vi "Test Executive.vi"() -> ()   [LabVIEW 2020]
uses:
  Library - Test Executive.llb/Test Executive - Globals.vi
panel:
  in  "Help":bool
  in  "Calibration":bool
  in  "Manual Control":bool
  in  "Sequence Tab":bool
  out "Abort":bool
  out "Error":bool
  out "Running":bool
  in  "Tab Control":enum32{"TS", "M", "C", "H"}(tab)
  in  "Comment":string
  in  "Serial Number":string
  out "Sequence":string
  out "Report Text":string
  in  "Operator":string
  in  "Save Report":bool
  in  "Clear Report Text":bool
  out "Sequence Name":string="None"
  in  "Abort Button":bool
  in  "Sequence Run":bool
  in  "Sequence Load":bool
  out "Help Text":string="This is some help text\n"
  in  "Quit":bool
  # "Sequence"
  # "Progress"
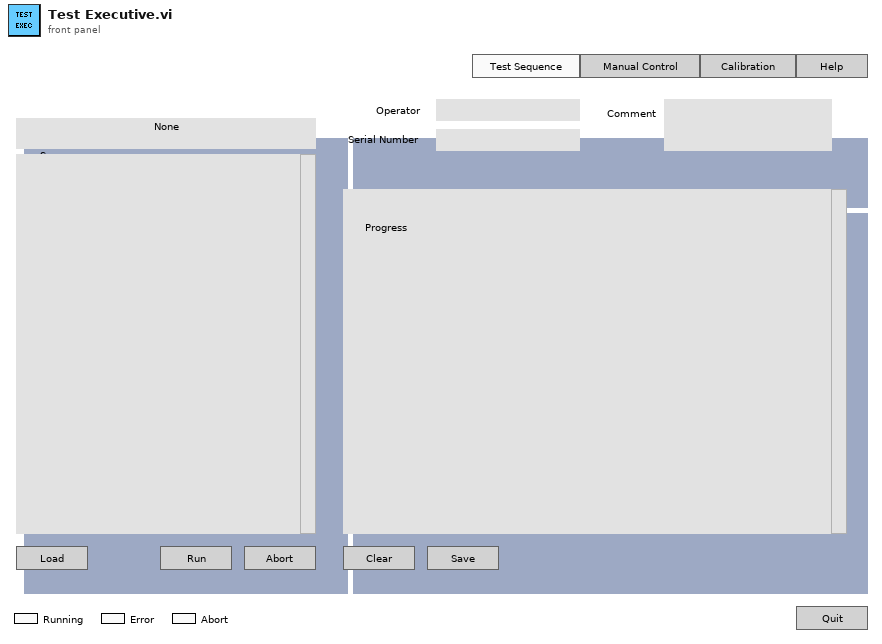
[diagram p1: front panel]
types:
  T1 = cluster{"Operator":string, "Serial Number":string, "Comment":string}
  T2 = cluster{"Operator Name":string, "UUT Serial Number":string, "Comment":string}
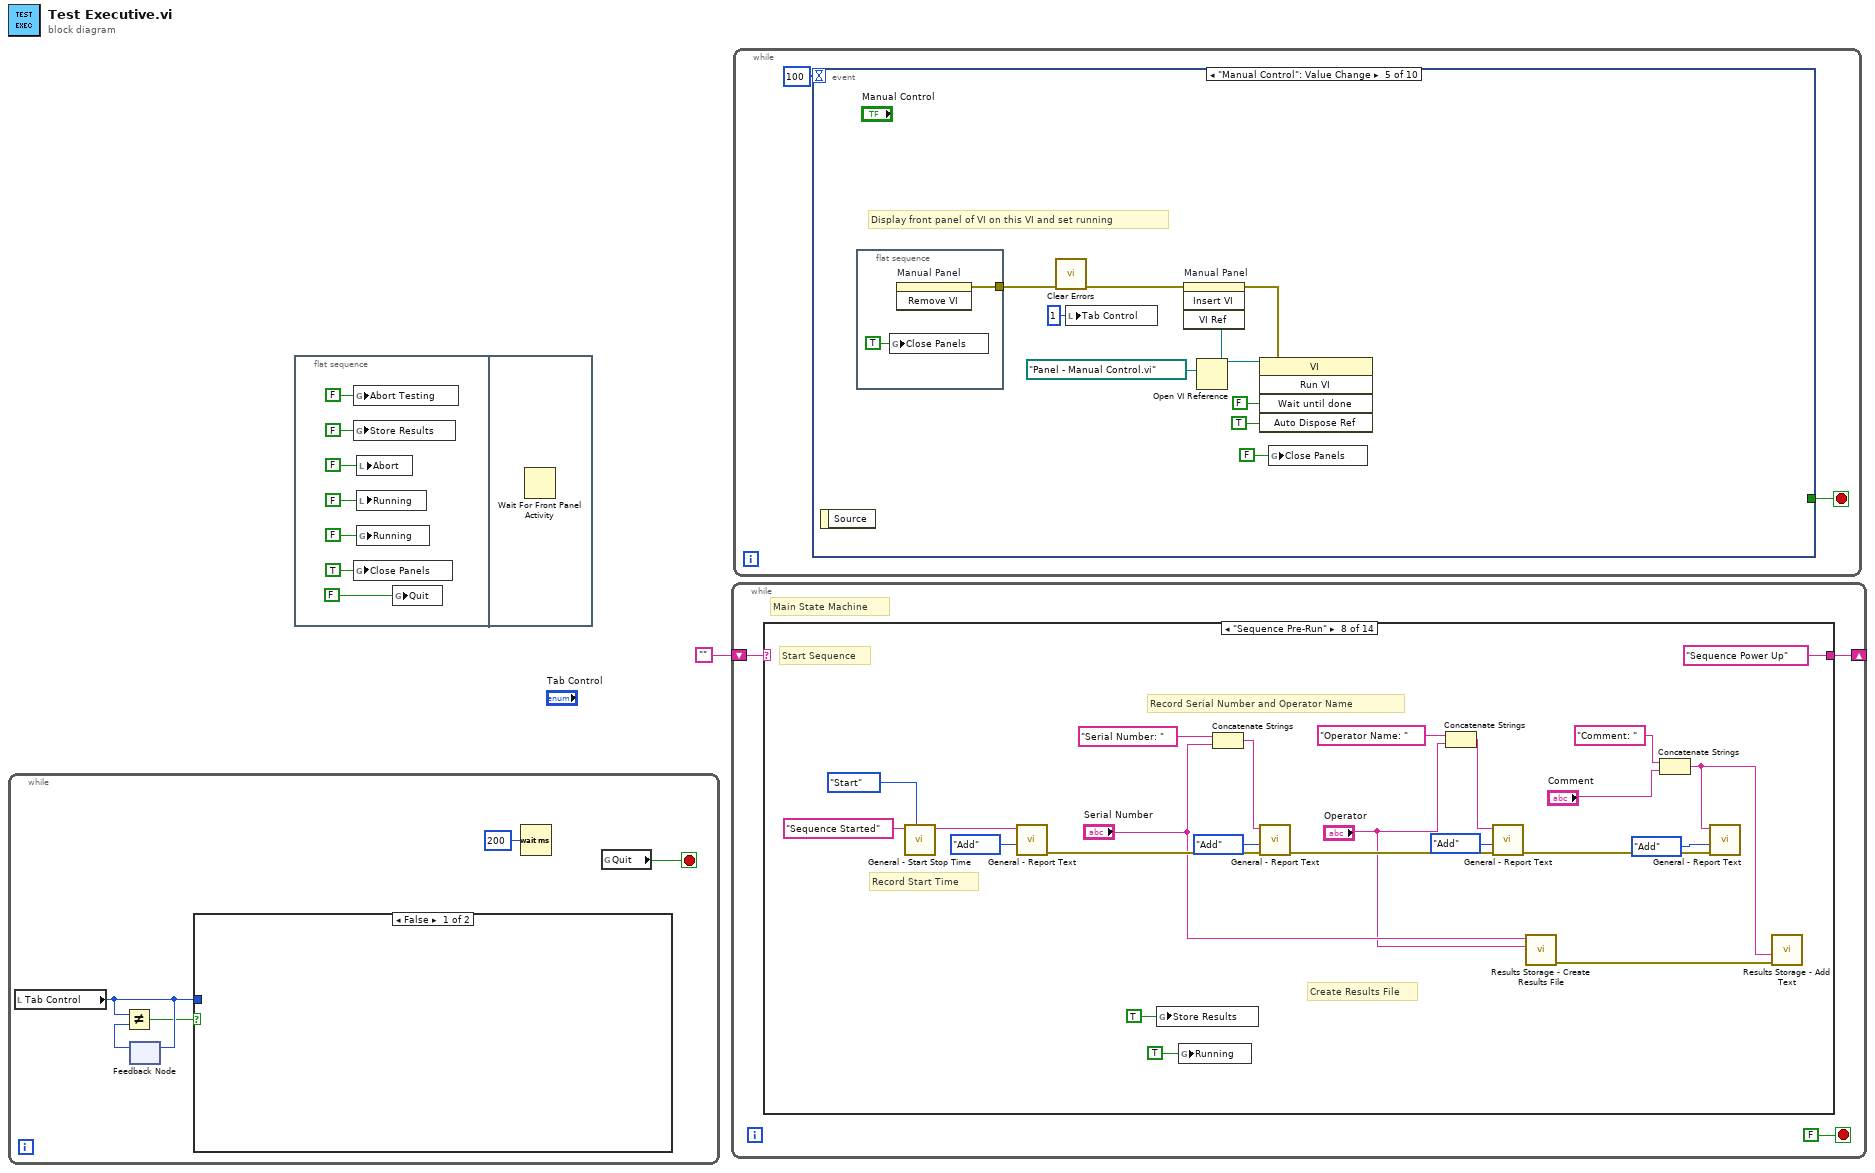
[diagram p0: block diagram]
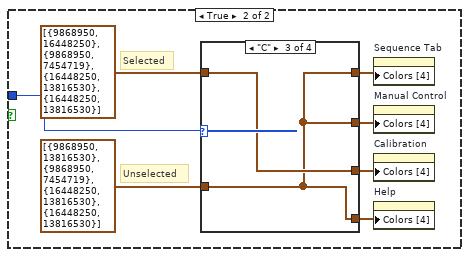
[diagram p2: hidden frame]
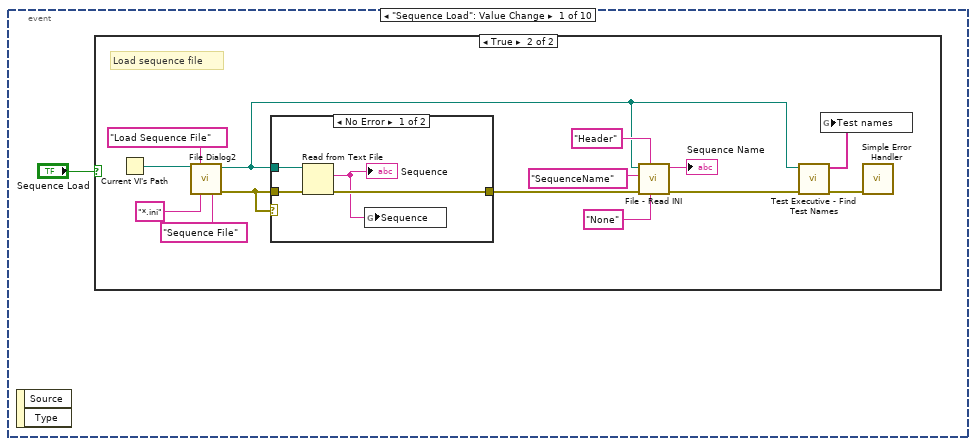
[diagram p6: hidden frame]
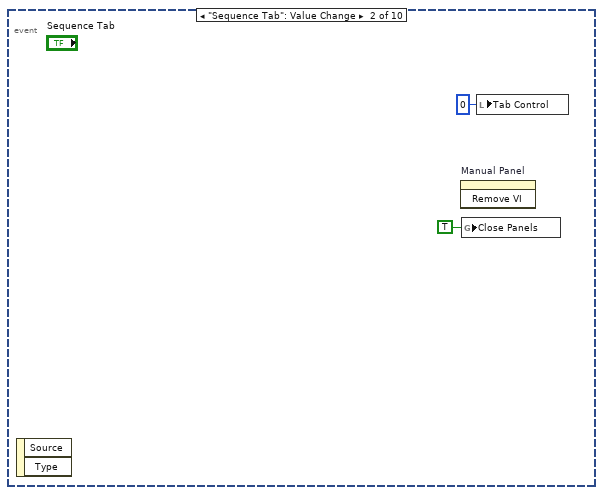
[diagram p9: hidden frame]
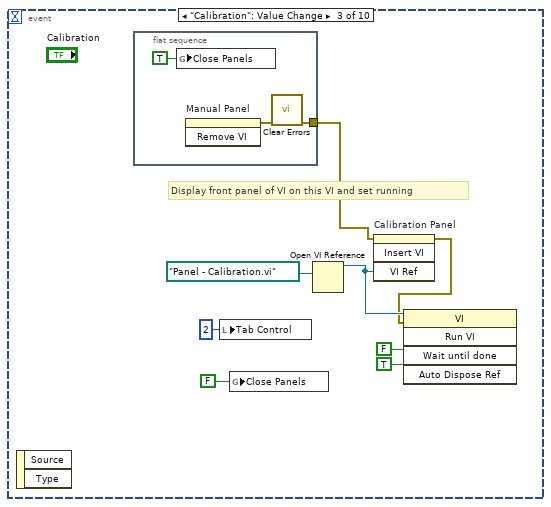
[diagram p10: hidden frame]
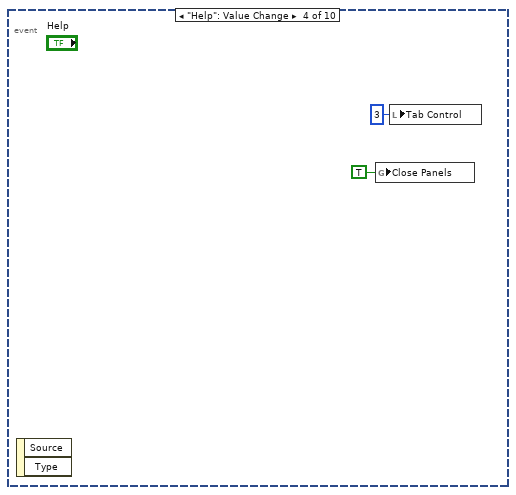
[diagram p11: hidden frame]
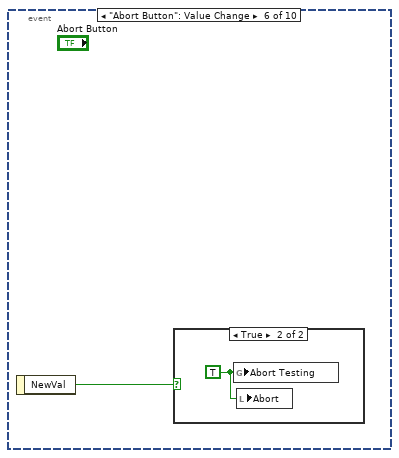
[diagram p12: hidden frame]
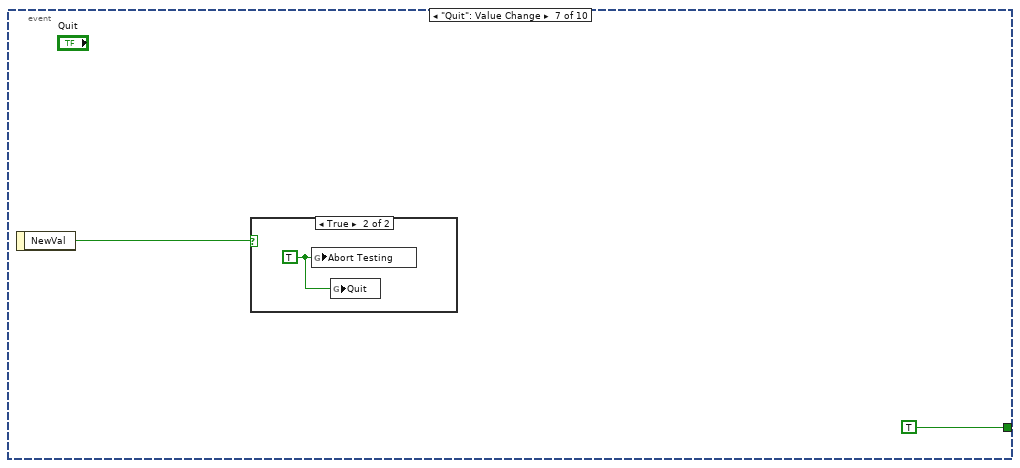
[diagram p14: hidden frame]
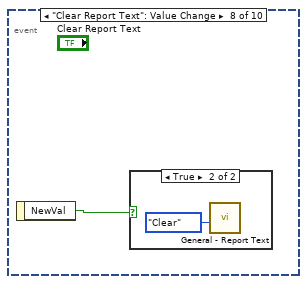
[diagram p16: hidden frame]
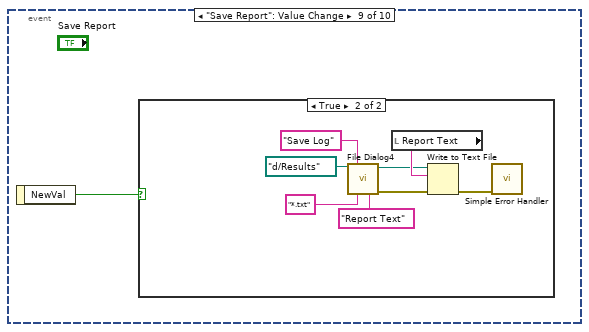
[diagram p18: hidden frame]
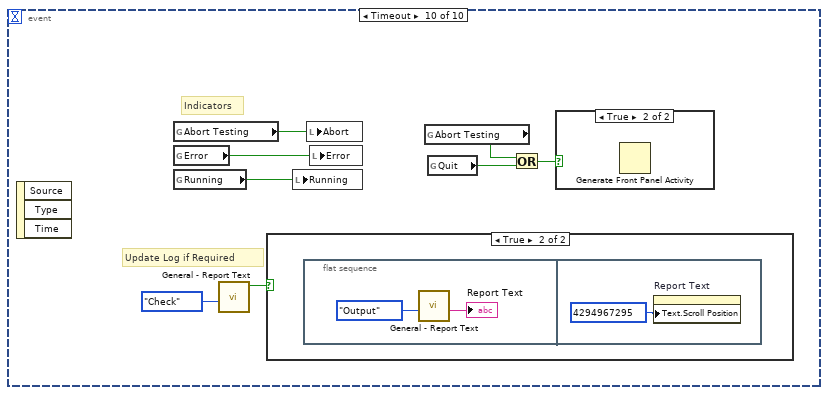
[diagram p20: hidden frame]
diagram:
  n1 = while {
    stop <- w3 stop-if-true
    n2 = local read "Tab Control"() -> (w6:enum32{"TS", "M", "C", "H"})
    n3 = feedback #1() -> (w4:enum32{"TS", "M", "C", "H"})  [unwired: 1 in]
    n4 = Not Equal?(x=w6, y=w4) -> (x != y?=w5:bool)
    n5 = feedback-in #1(w6) -> ()
    n6 = case shown="False" w5 {
      tunnel: w6 -> [_ w13]
      frame False {
      }
      frame True {
        # "Unselected"
        # "Selected"
        n7 = case shown="\"C\"" w13 {
          tunnel: cluster{u32, u32}[] [{9868950, 16448250}, {9868950, 7454719}, {16448250, 13816530}, {16448250, 13816530}] ("Colors [4]") -> [w15 w17 w19 w21]
          tunnel: cluster{u32, u32}[] [{9868950, 13816530}, {9868950, 7454719}, {16448250, 13816530}, {16448250, 13816530}] ("Colors [4]") -> [w14 w16 w18 w20]
          tunnel: [w15 w16 w18 w20] -> w10
          tunnel: [w14 w17 w18 w20] -> w9
          tunnel: [w14 w16 w19 w20] -> w8
          tunnel: [w14 w16 w18 w21] -> w7
          frame "TS", Default {
          }
          frame "M" {
          }
          frame "C" {
          }
          frame "H" {
          }
        }
        n8 = property on="Sequence Tab" class="Bool"("Colors [4]"=w10) -> ()  [unwired: 2 in, 2 out]
        n9 = property on="Manual Control" class="Bool"("Colors [4]"=w9) -> ()  [unwired: 2 in, 2 out]
        n10 = property on="Calibration" class="Bool"("Colors [4]"=w8) -> ()  [unwired: 2 in, 2 out]
        n11 = property on="Help" class="Bool"("Colors [4]"=w7) -> ()  [unwired: 2 in, 2 out]
      }
    }
    n12 = Wait (ms)(milliseconds to wait=u32 200) -> ()  [unwired: 1 out]
    n13 = global read "Test Executive - Globals.vi" "Quit"() -> (w3:bool)
  }
  n14 = flat-sequence {
    frame #0 {
      n15 = global write "Test Executive - Globals.vi" "Abort Testing"(FALSE ("Abort Testing")) -> ()
      n16 = global write "Test Executive - Globals.vi" "Store Results"(FALSE ("Abort Testing")) -> ()
      n17 = global write "Test Executive - Globals.vi" "Close Panels"(TRUE ("Close Panels")) -> ()
      n18 = local write "Abort"(FALSE ("Abort")) -> ()
      n19 = local write "Running"(FALSE ("Abort")) -> ()
      n20 = global write "Test Executive - Globals.vi" "Running"(FALSE ("Test Running")) -> ()
      n21 = global write "Test Executive - Globals.vi" "Quit"(FALSE ("Quit")) -> ()
    }
    frame #1 {
      n22 = Wait For Front Panel Activity() -> ()  [unwired: 3 in, 1 out]
    }
  }
  n23 = while {
    shift-right: [w30] -> _
    shift-left: "" -> [w31]
    stop <- FALSE stop-if-true
    # "Main State Machine"
    n24 = case shown="\"Sequence Pre-Run\"" w31 {
      tunnel: ["Idle" w58 w64 w65 w77 w115 "Sequence Pre-Run" ("f") "Sequence Power Up" ("f") "Sequence Running" ("f") "Sequence Power Down" ("f") "Sequence Pass Fail" ("f") "Sequence Store Results" ("f") "Idle" ("f") ""] -> w30
      frame "Start", Default {
        w34 = FALSE
        w35 = FALSE ("Running")
        # "Hide tab control (make transparent)"
        # "Auto Load Main Sequence"
        # "Load Help Text"
        # "Clear Indicators"
        # "Define File Paths"
        # "Define Test Equipment"
        n25 = disable-structure shown="Disabled" {
          frame Disabled {
            n26 = property class="VI" props=["Panel"]() -> (reference out=w46:refnum<vi>)  [unwired: 2 in, 2 out]
            n27 = call "Dialog Box - Resize Window.vi"("Height"=i16 493, "Width"=i16 900, "reference"=w46) -> ()  [unwired: 8 in, 1 out]
          }
          frame Enabled {
          }
        }
        n28 = call "Sequence - Define Test Equipment.vi"() -> ()  [unwired: 11 in, 1 out]
        n29 = global write "Test Executive - Globals.vi" "Abort Testing"(w34) -> ()
        n30 = global write "Test Executive - Globals.vi" "Error"(w34) -> ()
        n31 = global write "Test Executive - Globals.vi" "Running"(w34) -> ()
        n32 = global write "Test Executive - Globals.vi" "Quit"(w34) -> ()
        n33 = call "Test Executive - Define Paths.vi"() -> ()  [unwired: 12 in]
        n34 = call <vilib>:"Application Directory.vi"() -> ("Application Directory"=w36:path)
        n35 = property on="Tab Control" class="TabCtl (strict)"("Colors"=cluster{u32, u32} {16777216, 16777216}, "Tabs Visible?"=FALSE) -> ()  [unwired: 2 in, 2 out]
        n36 = Build Path(base path=w36, name or relative path="Help.txt") -> (appended path=w43:path)
        n37 = Build Path(base path=w36, name or relative path="Sequence - Main.ini") -> (appended path=w37:path)
        n38 = Read from Text File(file (use dialog)=w43) -> (text=w42:string, error out=w41:errorcluster)  [unwired: 3 in, 2 out]
        n39 = Read from Text File(file (use dialog)=w37) -> (text=w39:string, error out=w40:errorcluster)  [unwired: 3 in, 2 out]
        n40 = case shown="No Error" w41 {
          tunnel: w42 -> [w56 _]
          frame No Error {
            "Help Text" <- w56
          }
          frame Error {
          }
        }
        n41 = case shown="No Error" w40 {
          tunnel: w39 -> [w50 _]
          tunnel: w37 -> [w51 _]
          frame No Error {
            n42 = local write "Sequence"(w50) -> ()
            n43 = call "Test Executive - Find Test Names.vi"("Configuration File Path"=w51) -> ("Test Names"=w49:string[])  [unwired: 9 in, 1 out]
            n44 = global write "Test Executive - Globals.vi" "Test names"(w49) -> ()
            n45 = call "File - Read INI.vi"("Default String"="None", "Section"="Header", "Key"="SequenceName", "configuration file path"=w51) -> ("String"=w52:string)  [unwired: 6 in, 1 out]
            n46 = local write "Sequence Name"(w52) -> ()
            n47 = global write "Test Executive - Globals.vi" "Sequence"(w50) -> ()
          }
          frame Error {
          }
        }
        "Running" <- w35
        "Error" <- w35
        "Abort" <- w35
      }
      frame "Idle" {
        # "Wait For Front Panel Activity"
        n48 = global read "Test Executive - Globals.vi" "Quit"() -> (w60:bool)
        n49 = Select(t="Quit", s=w60, f="Sequence Controls") -> (s? t:f=w58:string)
      }
      frame "Sequence Controls" {
        # "Sequence Controls"
        n50 = Select(t="Sequence Check", s="Sequence Run", f="Idle") -> (s? t:f=w64:string)
      }
      frame "Sequence Check" {
        # "Check Sequence Name"
        # "Sequence Check"
        n51 = local read "Sequence Name"() -> (w67:string)
        n52 = Equal?(x=w67, y="None") -> (x = y?=w69:bool)
        n53 = case shown="True" w69 {
          tunnel: "Sequence Start" -> [w70 _]
          tunnel: [w70 "Idle"] -> w65
          frame False {
          }
          frame True {
            n54 = call "Dialog Box - One Button.vi"("Text"="ERROR: Sequence name is set to \"None\".") -> ()  [unwired: 10 in, 1 out]
          }
        }
      }
      frame "Sequence Start" {
        # "Start of Sequence"
        # "Configure Results Storage"
        n55 = local read "Serial Number"() -> (w87:string)
        n56 = call <vilib>:"Dflt Data Dir.vi"() -> ("App:Default Data Directory"=w90:path)
        n57 = local read "Comment"() -> (w85:string)
        n58 = local read "Operator"() -> (w88:string)
        n59 = Build Path(base path=w90, name or relative path="Results") -> (appended path=w91:path)
        n60 = call "General - Check if Mac.vi"() -> ("Mac"=w92:bool)  [unwired: 2 in]
        n61 = Path To String(path=w91) -> (string=w75:string)
        n62 = Bundle("Operator"=w88, "Serial Number"=w87, "Comment"=w85) -> (w86:T1)  [unwired: 1 in]
        n63 = case shown="False" w92 {
          tunnel: [w109 w113] -> w73
          tunnel: w75 -> [w107 w111]
          frame True {
            n64 = call "Test Executive - Sequence File Value.vi"("Default String"=w107, "Section (Current Test)"="results" ("Section"), "Key"="directorymac") -> ("String"=w109:string)  [unwired: 5 in, 3 out]
          }
          frame False {
            n65 = call "Test Executive - Sequence File Value.vi"("Default String"=w111, "Section (Current Test)"="results" ("Section"), "Key"="directorywin") -> ("String"=w113:string)  [unwired: 5 in, 3 out]
          }
        }
        n66 = disable-structure shown="Enabled" {
          disable-tunnel: w86 -> [w100 _]
          disable-tunnel: [w99 _] -> w84
          disable-tunnel: [w98 FALSE ("Cancel")] -> w78
          frame Disabled {
            n67 = call "Dialog Box - Test Details.vi"("Values In"=w100) -> ("Values Out"=w99:T2, "Cancel"=w98:bool)  [unwired: 7 in, 1 out]
          }
          frame Enabled {
          }
        }
        n68 = Unbundle By Name(w84) -> ("Operator Name"=w83:string, "UUT Serial Number"=w82:string, "Comment"=w81:string)
        n69 = call "General - Check if Linux.vi"() -> ("Linux"=w76:bool)  [unwired: 2 in]
        n70 = case shown="False" w76 {
          tunnel: [w104 w106] -> w74
          tunnel: w75 -> [w102 _]
          tunnel: w73 -> [_ w106]
          frame True {
            n71 = call "Test Executive - Sequence File Value.vi"("Default String"=w102, "Section (Current Test)"="results" ("Section"), "Key"="directorylinux") -> ("String"=w104:string)  [unwired: 5 in, 3 out]
          }
          frame False {
          }
        }
        n72 = local write "Serial Number"(w82) -> ()
        n73 = local write "Operator"(w83) -> ()
        n74 = local write "Comment"(w81) -> ()
        n75 = String To Path(string=w74) -> (path=w94:path)
        n76 = global write "Test Executive - Globals.vi" "Operator Name"(w83) -> ()
        n77 = global write "Test Executive - Globals.vi" "Serial Number"(w82) -> ()
        n78 = global write "Test Executive - Globals.vi" "Comment"(w81) -> ()
        n79 = global write "Test Executive - Globals.vi" "Results Directory"(w94) -> ()
        n80 = call "Results Storage - Setup.vi"("Rename Files on Close"=TRUE, "Results Directory"=w94) -> ()  [unwired: 9 in, 1 out]
        n81 = call "General - Report Text.vi"("Mode (Add)"=enum16{"Add", "Output", "Clear", "Check"}."Clear") -> ()  [unwired: 8 in, 3 out]
        n82 = global write "Test Executive - Globals.vi" "Abort Testing"(FALSE ("Abort Testing")) -> ()
        n83 = global write "Test Executive - Globals.vi" "Unit Passed"(FALSE ("Pass")) -> ()
        n84 = Select(t="Idle" ("f"), s=w78, f="Sequence Check Equipment") -> (s? t:f=w77:string)
      }
      frame "Sequence Check Equipment" {
        # "Check Test Equipment"
        # "Check Test Equipment"
        n85 = call "Sequence - Check Test Equipment.vi"() -> ("error out"=w118:errorcluster, "PASS"=w119:bool)  [unwired: 10 in]
        n86 = Not(x=w119) -> (.not. x?=w117:bool)
        n87 = case shown="False" w117 {
          tunnel: "Sequence Asset" -> [w120 _]
          tunnel: [w120 "Idle"] -> w115
          tunnel: w118 -> [_ _]
          frame False {
          }
          frame True {
            n88 = call "Dialog Box - One Button.vi"("Text"="ERROR: Test equipment check failed.") -> ()  [unwired: 10 in, 1 out]
          }
        }
      }
      frame "Sequence Asset" {
        # "Test Equipment is Defined is \"Sequence - Define Test Equipment.vi\""
        # "Enter Equipment Asset Numbers"
        n89 = global read "Test Executive - Globals.vi" "Asset Number Recording"() -> (w123:bool)
        n90 = case shown="True" w123 {
          frame False {
          }
          frame True {
            n91 = call "Test Equipment - Asset Numbers.vi"("Mode"=enum16{"Edit", "Define", "Load", "Save", "CSV"}."Load") -> ("error out"=w125:errorcluster)  [unwired: 9 in, 1 out]
            n92 = call "Test Equipment - Asset Numbers.vi"("error in (no error)"=w125, "Mode"=enum16{"Edit", "Define", "Load", "Save", "CSV"}."Edit") -> ("error out"=w126:errorcluster)  [unwired: 8 in, 1 out]
            n93 = call "Test Equipment - Asset Numbers.vi"("error in (no error)"=w126, "Mode"=enum16{"Edit", "Define", "Load", "Save", "CSV"}."Save") -> ()  [unwired: 8 in, 2 out]
          }
        }
      }
      frame "Sequence Pre-Run" {
        # "Create Results File"
        # "Record Serial Number and Operator Name"
        # "Record Start Time"
        # "Start Sequence"
        n94 = call "General - Start Stop Time.vi"("Start / Stop (Start)"=enum16{"Start", "Stop"}."Start", "Initial String"="Sequence Started") -> ("String with Time / Date"=w150:string)  [unwired: 8 in, 1 out]
        n95 = call "General - Report Text.vi"("Mode (Add)"=enum16{"Add", "Output", "Clear", "Check"}."Add", "Text In"=w150) -> ("error out"=w141:errorcluster)  [unwired: 7 in, 2 out]
        n96 = global write "Test Executive - Globals.vi" "Store Results"(TRUE ("Store Results")) -> ()
        n97 = global write "Test Executive - Globals.vi" "Running"(TRUE ("Test Running")) -> ()
        n98 = Concatenate Strings("Serial Number: " ("string"), "Serial Number") -> (w146:string)
        n99 = call "General - Report Text.vi"("error in (no error)"=w141, "Mode (Add)"=enum16{"Add", "Output", "Clear", "Check"}."Add", "Text In"=w146) -> ("error out"=w140:errorcluster)  [unwired: 6 in, 2 out]
        n100 = Concatenate Strings("Operator Name: " ("string"), "Operator") -> (w143:string)
        n101 = call "General - Report Text.vi"("error in (no error)"=w140, "Mode (Add)"=enum16{"Add", "Output", "Clear", "Check"}."Add", "Text In"=w143) -> ("error out"=w132:errorcluster)  [unwired: 6 in, 2 out]
        n102 = call "Results Storage - Create Results File.vi"("Operator Name"="Operator", "Serial Number"="Serial Number") -> ("error out"=w131:errorcluster)  [unwired: 9 in]
        n103 = Concatenate Strings("Comment: " ("string"), "Comment") -> (w130:string)
        n104 = call "General - Report Text.vi"("error in (no error)"=w132, "Mode (Add)"=enum16{"Add", "Output", "Clear", "Check"}."Add", "Text In"=w130) -> ()  [unwired: 6 in, 3 out]
        n105 = call "Results Storage - Add Text.vi"("error in (no error)"=w131, "Text"=w130) -> ()  [unwired: 9 in, 1 out]
      }
      frame "Sequence Power Up" {
        # "Reset all Test Equipment then Power Up Unit Under Test"
        # "Sequence Power Up"
        n106 = call "Sequence - Reset All.vi"() -> ("error out"=w157:errorcluster)  [unwired: 11 in]
        n107 = call "Test Executive - Display Error.vi"("Clear Error"=TRUE, "error in (no error)"=w157) -> ("error out"=w156:errorcluster)  [unwired: 9 in]
        n108 = call "Sequence - Power Up.vi"("error in (no error)"=w156) -> ("error out"=w155:errorcluster)  [unwired: 10 in]
        n109 = call "Test Executive - Display Error.vi"("Clear Error"=TRUE, "error in (no error)"=w155) -> ()  [unwired: 9 in, 1 out]
      }
      frame "Sequence Running" {
        # "Run Sequence"
        n110 = global read "Test Executive - Globals.vi" "Test names"() -> (w159:string[])
        n111 = for {
          tunnel: w159 -> [w162] mode=indexing
          stop <- w163 stop-if-true
          # "Step Through Each Test"
          n112 = call "Sequence - Action Test.vi"("Test"=w162) -> ("error out"=w161:errorcluster)  [unwired: 10 in]
          n113 = stacked-sequence {
            tunnel: [w166] -> w163
            tunnel: w161 -> [w165]
            frame #0 {
              n114 = call "Test Executive - Display Error.vi"("error in (no error)"=w165) -> ("error out"=w164:errorcluster)  [unwired: 10 in]
              n115 = Unbundle By Name(w164) -> ("status"=w167:bool)
              n116 = global read "Test Executive - Globals.vi" "Abort Testing"() -> (w166:bool)
              n117 = local write "Error"(w167) -> ()
            }
          }
        }
      }
      frame "Sequence Power Down" {
        # "Power Down Unit Under Test then Reset all Test Equipment"
        # "Sequence Power Down"
        n118 = call "Sequence - Power Down.vi"() -> ("error out"=w168:errorcluster)  [unwired: 11 in]
        n119 = call "Test Executive - Display Error.vi"("Clear Error"=TRUE, "error in (no error)"=w168) -> ("error out"=w169:errorcluster)  [unwired: 9 in]
        n120 = call "Sequence - Reset All.vi"("error in (no error)"=w169) -> ("error out"=w170:errorcluster)  [unwired: 10 in]
        n121 = call "Test Executive - Display Error.vi"("Clear Error"=TRUE, "error in (no error)"=w170) -> ()  [unwired: 9 in, 1 out]
      }
      frame "Sequence Pass Fail" {
        # "Add Stop Time"
        # "Sequence Pass / Fail"
        # "Display Banner"
        # "Pass / Fail ??"
        n122 = call "General - Report Text.vi"("Mode (Add)"=enum16{"Add", "Output", "Clear", "Check"}."Output") -> ("Report Text Out"=w183:string)  [unwired: 8 in, 2 out]
        n123 = Search/Split String(string=w183, search string/char (-)="ERROR") -> (offset of match=w203:i32)  [unwired: 1 in, 2 out]
        n124 = Search/Split String(string=w183, search string/char (-)="FAIL") -> (offset of match=w197:i32)  [unwired: 1 in, 2 out]
        n125 = Search/Split String(string=w183, search string/char (-)="PASS") -> (offset of match=w184:i32)  [unwired: 1 in, 2 out]
        n126 = Greater Than 0?(x=w203) -> (x > 0?=w204:bool)
        n127 = Greater Than 0?(x=w197) -> (x > 0?=w198:bool)
        n128 = Greater Than 0?(x=w184) -> (x > 0?=w181:bool)
        n129 = Select(t="UNIT PASSED", s=w181, f="UNIT FAILED") -> (s? t:f=w180:string)
        n130 = Select(t="UNIT FAILED", s=w198, f=w180) -> (s? t:f=w205:string)
        n131 = global read "Test Executive - Globals.vi" "Abort Testing"() -> (w175:bool)
        n132 = Select(t="UNIT FAILED (ERRORS)", s=w204, f=w205) -> (s? t:f=w178:string)
        n133 = Select(t="TESTING ABORTED", s=w175, f=w178) -> (s? t:f=w176:string)
        n134 = Select(t="Sequence Aborted", s=w175, f="Sequence Completed" ("Initial String")) -> (s? t:f=w192:string)
        n135 = call "General - Report Text.vi"("Mode (Add)"=enum16{"Add", "Output", "Clear", "Check"}."Add", "Text In"=w176) -> ("error out"=w188:errorcluster)  [unwired: 7 in, 2 out]
        n136 = call "General - Start Stop Time.vi"("Start / Stop (Start)"=enum16{"Start", "Stop"}."Stop", "Initial String"=w192) -> ("String with Time / Date"=w190:string)  [unwired: 8 in, 1 out]
        n137 = Equal?(x="UNIT PASSED", y=w176) -> (x = y?=w174:bool)
        n138 = global write "Test Executive - Globals.vi" "Unit Passed"(w174) -> ()
        n139 = call "Dialog Box - Pass Fail Banner.vi"("Pass"=w174, "Text"=w176) -> ()  [unwired: 9 in, 1 out]
        n140 = call "General - Report Text.vi"("error in (no error)"=w188, "Mode (Add)"=enum16{"Add", "Output", "Clear", "Check"}."Add", "Text In"=w190) -> ()  [unwired: 6 in, 3 out]
      }
      frame "Sequence Store Results" {
        # "Record Asset Numbers"
        # "Sequence Store Results"
        # "Close Results File"
        n141 = global read "Test Executive - Globals.vi" "Asset Number Recording"() -> (w209:bool)
        n142 = global read "Test Executive - Globals.vi" "Unit Passed"() -> (w206:bool)
        n143 = case shown="True" w209 {
          tunnel: [_ w217] -> w208
          frame False {
          }
          frame True {
            n144 = call "Test Equipment - Asset Numbers.vi"("Mode"=enum16{"Edit", "Define", "Load", "Save", "CSV"}."CSV") -> ("Output"=w218:string)  [unwired: 9 in, 1 out]
            n145 = call "Results Storage - Add Text.vi"("Add New Line (True)"=FALSE, "Text"=w218) -> ("error out"=w217:errorcluster)  [unwired: 9 in]
          }
        }
        n146 = global read "Test Executive - Globals.vi" "Abort Testing"() -> (w207:bool)
        n147 = Select(t=enum16{"auto", "passed", "failed", "aborted"}."passed" ("Result (auto)"), s=w206, f=enum16{"auto", "passed", "failed", "aborted"}."failed" ("Result (auto)")) -> (s? t:f=w211:enum16{"auto", "passed", "failed", "aborted"})
        n148 = Select(t=enum16{"auto", "passed", "failed", "aborted"}."aborted" ("Result (auto)"), s=w207, f=w211) -> (s? t:f=w210:enum16{"auto", "passed", "failed", "aborted"})
        n149 = call "Results Storage - Close Results File.vi"("error in (no error)"=w208, "Result (auto)"=w210) -> ()  [unwired: 9 in, 1 out]
      }
      frame "Quit" {
        # "Exit Program"
        n150 = flat-sequence {
          frame #0 {
            # "Exit completely if\ncompiled"
            n151 = call "General - Check if EXE.vi"() -> ("EXE"=w221:bool)  [unwired: 2 in]
            n152 = global write "Test Executive - Globals.vi" "Close Panels"(TRUE ("Close Panels")) -> ()
            n153 = Quit LabVIEW(quit? (T)=w221) -> ()
          }
          frame #1 {
            # "Make tab control visible"
            n154 = property on="Tab Control" class="TabCtl (strict)"("Colors"=cluster{u32, u32} {7171459, 7171459}, "Tabs Visible?"=TRUE) -> ()  [unwired: 2 in, 2 out]
          }
          frame #2 {
            n155 = Stop() -> ()  [unwired: 1 in]
          }
        }
      }
    }
  }
  n156 = while {
    stop <- w225 stop-if-true
    n157 = event shown="[4] \"Manual Control\": Value Change" {
      selector: _ -> [_ _ _ _ _ _ _ _ _ _]
      dyn-events: _ -> [_ _ _ _ _ _ _ _ _ _]
      timeout: 100 -> [_ _ _ _ _ _ _ _ _ _]
      tunnel: [_ _ _ _ _ _ TRUE _ _ _] -> w225
      event "Sequence Load": Value Change {
        n158 = event-data() -> ()  [unwired: 1 in, 2 out]
        n159 = case shown="True" "Sequence Load" {
          frame False {
          }
          frame True {
            # "Load sequence file"
            n160 = Current VI's Path() -> (path=w239:path)
            n161 = call "File Dialog2"("start path"=w239, "prompt"="Load Sequence File", "pattern (all files)"="*.ini", "pattern label"="Sequence File") -> ("selected path"=w231:path, "error out"=w237:errorcluster)  [unwired: 8 in, 2 out]
            n162 = case shown="No Error" w237 {
              tunnel: w237 -> [w245 w246]
              tunnel: w231 -> [w244 _]
              tunnel: [w243 w246] -> w233
              frame No Error {
                n163 = Read from Text File(file (use dialog)=w244, error in=w245) -> (text=w242:string, error out=w243:errorcluster)  [unwired: 2 in, 2 out]
                "Sequence" <- w242
                n164 = global write "Test Executive - Globals.vi" "Sequence"(w242) -> ()
              }
              frame Error {
              }
            }
            n165 = call "File - Read INI.vi"("Default String"="None", "Section"="Header", "error in (no error)"=w233, "Key"="SequenceName", "configuration file path"=w231) -> ("error out"=w230:errorcluster, "String"=→"Sequence Name":string)  [unwired: 5 in]
            n166 = call "Test Executive - Find Test Names.vi"("error in (no error)"=w230, "Configuration File Path"=w231) -> ("error out"=w229:errorcluster, "Test Names"=w228:string[])  [unwired: 8 in]
            n167 = global write "Test Executive - Globals.vi" "Test names"(w228) -> ()
            n168 = call <vilib>:"Simple Error Handler.vi"("error in (no error)"=w229) -> ()  [unwired: 4 in, 5 out]
          }
        }
      }
      event "Sequence Tab": Value Change {
        n169 = event-data() -> ()  [unwired: 1 in, 2 out]
        n170 = invoke on="Manual Panel" class="SubPanel" method="Remove VI"() -> ()  [unwired: 3 in, 3 out]
        n171 = global write "Test Executive - Globals.vi" "Close Panels"(TRUE ("Close Panels")) -> ()
        n172 = local write "Tab Control"(u8 0) -> ()
      }
      event "Calibration": Value Change {
        # "Display front panel of VI on this VI and set running"
        n173 = event-data() -> ()  [unwired: 1 in, 2 out]
        n174 = flat-sequence {
          tunnel: [w258] -> w249
          frame #0 {
            n175 = global write "Test Executive - Globals.vi" "Close Panels"(TRUE ("Close Panels")) -> ()
            n176 = invoke on="Manual Panel" class="SubPanel" method="Remove VI"() -> (error out=w259:errorcluster)  [unwired: 3 in, 2 out]
            n177 = call <vilib>:"Clear Errors.vi"("error in (no error)"=w259) -> ("error out"=w258:errorcluster)  [unwired: 5 in, 1 out]
          }
        }
        n178 = local write "Tab Control"(u8 2) -> ()
        n179 = global write "Test Executive - Globals.vi" "Close Panels"(FALSE ("Close Panels")) -> ()
        n180 = Open VI Reference(vi path=path "Panel - Calibration.vi") -> (vi reference=w255:refnum<vi>)  [unwired: 5 in, 1 out]
        n181 = invoke on="Calibration Panel" class="SubPnl" method="Insert VI"(error in=w249, "VI Ref"=w255) -> (error out=w254:errorcluster)  [unwired: 2 in, 3 out]
        n182 = invoke class="VI" method="Run VI"(reference=w255, error in=w254, "Wait until done"=FALSE ("Wait Until Done"), "Auto Dispose Ref"=TRUE ("Auto Dispose Reference")) -> ()  [unwired: 1 in, 5 out]
      }
      event "Help": Value Change {
        n183 = event-data() -> ()  [unwired: 1 in, 2 out]
        n184 = global write "Test Executive - Globals.vi" "Close Panels"(TRUE ("Close Panels")) -> ()
        n185 = local write "Tab Control"(u8 3) -> ()
      }
      event "Manual Control": Value Change {
        # "Display front panel of VI on this VI and set running"
        n186 = event-data() -> ()  [unwired: 1 in, 1 out]
        n187 = flat-sequence {
          tunnel: [w272] -> w263
          frame #0 {
            n188 = global write "Test Executive - Globals.vi" "Close Panels"(TRUE ("Close Panels")) -> ()
            n189 = invoke on="Manual Panel" class="SubPanel" method="Remove VI"() -> (error out=w272:errorcluster)  [unwired: 3 in, 2 out]
          }
        }
        n190 = call <vilib>:"Clear Errors.vi"("error in (no error)"=w263) -> ("error out"=w262:errorcluster)  [unwired: 5 in, 1 out]
        n191 = local write "Tab Control"(u8 1) -> ()
        n192 = Open VI Reference(vi path=path "Panel - Manual Control.vi") -> (vi reference=w269:refnum<vi>)  [unwired: 5 in, 1 out]
        n193 = invoke on="Manual Panel" class="SubPanel" method="Insert VI"(error in=w262, "VI Ref"=w269) -> (error out=w268:errorcluster)  [unwired: 2 in, 3 out]
        n194 = invoke class="VI" method="Run VI"(reference=w269, error in=w268, "Wait until done"=FALSE ("Wait Until Done"), "Auto Dispose Ref"=TRUE ("Auto Dispose Reference")) -> ()  [unwired: 1 in, 5 out]
        n195 = global write "Test Executive - Globals.vi" "Close Panels"(FALSE ("Close Panels")) -> ()
      }
      event "Abort Button": Value Change {
        n196 = event-data() -> ("NewVal"=w273:bool)  [unwired: 1 in]
        n197 = case shown="True" w273 {
          frame False {
          }
          frame True {
            w274 = TRUE ("Abort Testing")
            n198 = global write "Test Executive - Globals.vi" "Abort Testing"(w274) -> ()
            n199 = local write "Abort"(w274) -> ()
          }
        }
      }
      event "Quit": Value Change {
        n200 = event-data() -> ("NewVal"=w276:bool)  [unwired: 1 in]
        n201 = case shown="True" w276 {
          frame False {
          }
          frame True {
            w277 = TRUE ("Abort Testing")
            n202 = global write "Test Executive - Globals.vi" "Abort Testing"(w277) -> ()
            n203 = global write "Test Executive - Globals.vi" "Quit"(w277) -> ()
          }
        }
      }
      event "Clear Report Text": Value Change {
        n204 = event-data() -> ("NewVal"=w278:bool)  [unwired: 1 in]
        n205 = case shown="True" w278 {
          frame False {
          }
          frame True {
            n206 = call "General - Report Text.vi"("Mode (Add)"=enum16{"Add", "Output", "Clear", "Check"}."Clear") -> ()  [unwired: 8 in, 3 out]
          }
        }
      }
      event "Save Report": Value Change {
        n207 = event-data() -> ("NewVal"=w280:bool)  [unwired: 1 in]
        n208 = case shown="True" w280 {
          frame False {
          }
          frame True {
            n209 = call "File Dialog4"("start path"=path "d:/Results", "prompt"="Save Log", "pattern (all files)"="*.txt", "pattern label"="Report Text") -> ("selected path"=w281:path, "error out"=w287:errorcluster)  [unwired: 8 in, 2 out]
            n210 = local read "Report Text"() -> (w286:string)
            n211 = Write to Text File(file (use dialog)=w281, text=w286, error in=w287) -> (error out=w288:errorcluster)  [unwired: 1 in, 2 out]
            n212 = call <vilib>:"Simple Error Handler.vi"("error in (no error)"=w288) -> ()  [unwired: 4 in, 5 out]
          }
        }
      }
      event Timeout {
        # "Indicators"
        # "Update Log if Required"
        n213 = event-data() -> ()  [unwired: 1 in, 3 out]
        n214 = global read "Test Executive - Globals.vi" "Abort Testing"() -> (w294:bool)
        n215 = global read "Test Executive - Globals.vi" "Error"() -> (w293:bool)
        n216 = global read "Test Executive - Globals.vi" "Running"() -> (w292:bool)
        n217 = call "General - Report Text.vi"("Mode (Add)"=enum16{"Add", "Output", "Clear", "Check"}."Check") -> ("Changed Out"=w296:bool)  [unwired: 8 in, 2 out]
        n218 = case shown="True" w296 {
          frame False {
          }
          frame True {
            n219 = flat-sequence {
              frame #0 {
                n220 = call "General - Report Text.vi"("Mode (Add)"=enum16{"Add", "Output", "Clear", "Check"}."Output") -> ("Report Text Out"=→"Report Text":string)  [unwired: 8 in, 2 out]
              }
              frame #1 {
                n221 = property on="Report Text" class="Str"("Text.Scroll Position"=u32 4294967295) -> ()  [unwired: 2 in, 2 out]
              }
            }
          }
        }
        n222 = local write "Running"(w292) -> ()
        n223 = local write "Abort"(w294) -> ()
        n224 = local write "Error"(w293) -> ()
        n225 = global read "Test Executive - Globals.vi" "Abort Testing"() -> (w289:bool)
        n226 = global read "Test Executive - Globals.vi" "Quit"() -> (w290:bool)
        n227 = Or(x=w289, y=w290) -> (x .or. y?=w291:bool)
        n228 = case shown="True" w291 {
          frame False {
          }
          frame True {
            n229 = Generate Front Panel Activity() -> ()  [unwired: 1 in]
          }
        }
      }
    }
  }
